vi "6.vi"() -> ()   [LabVIEW 2017]
panel:
  out "平均数":dbl
  out "最小值":dbl
  out "最大值":dbl
  out "波形图":dbl[](graph)
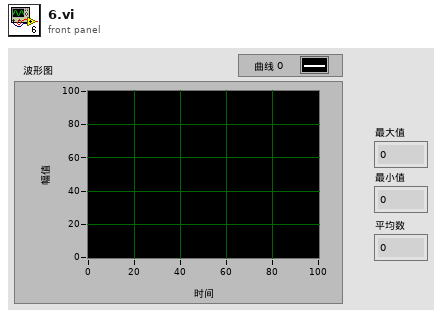
[diagram p1: front panel]
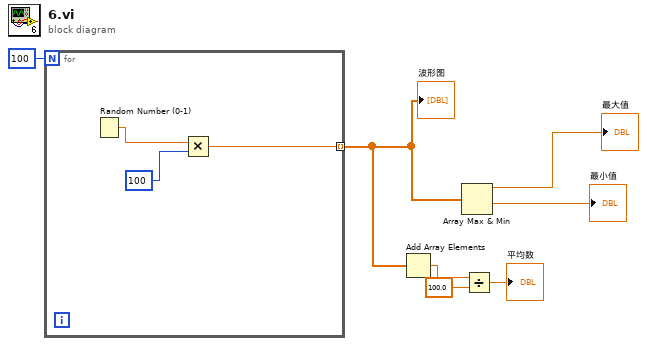
[diagram p0: block diagram]
diagram:
  n1 = for {
    N: 100 -> [_]
    tunnel: [w8] -> w4 mode=indexing
    n2 = Random Number (0-1)() -> (number: 0 to 1=w10:dbl)
    n3 = Multiply(x=w10, y=100) -> (x*y=w8:dbl)
  }
  "波形图" <- w4
  n4 = Add Array Elements(numeric array=w4) -> (sum=w3:dbl)
  n5 = Array Max & Min(array=w4) -> (max value=→"最大值":dbl, min value=→"最小值":dbl)  [unwired: 2 out]
  n6 = Divide(x=w3, y=100.0) -> (x/y=→"平均数":dbl)
